vi "Ass IO Status.vi"(8 "error in (no error)":errorcluster) -> (0 "error out":errorcluster)   [LabVIEW 2017]
uses:
  <vilib>/NI/Modbus Library/API/Wrapper/Create TCP Master.vi
  <vilib>/NI/Modbus Library/API/master/Modbus Master.lvclass
  <vilib>/NI/Modbus Library/API/Wrapper/API Main.lvlib
panel:
  in  "Tab Control":enum32{"INPUTS", "OUTPUTS"}(tab)
  out "Cycle Start-1":bool
  out "Cycle Start-2":bool
  out "Reset":bool
  out "Emergency":bool
  out "Bin-1":bool
  out "Bin-2":bool
  out "Bin-3":bool
  out "Bin-4":bool
  out "Bin-5":bool
  out "Bin-6":bool
  out "Bin-7":bool
  out "Bin-8":bool
  out "Part Presence":bool
  out "OK Cam-1":bool
  out "NOK Cam-1":bool
  out "OK Cam-2":bool
  out "NOK Cam-2":bool
  out "Part Clamp Fwd":bool
  out "Part Clamp Rev":bool
  in  "Red Tower Lamp":bool
  in  "Buzzer Tower Lamp":bool
  in  "Yellow Tower Lamp":bool
  in  "Green Tower Lamp":bool
  in  "Orange Ind Bin-01":bool
  in  "Yellow Ind Bin-01":bool
  in  "Green Ind Bin-01":bool
  in  "Orange Ind Bin-02":bool
  in  "Yellow Ind Bin-02":bool
  in  "Green Ind Bin-02":bool
  in  "Yellow Ind Bin-03":bool
  in  "Green Ind Bin-03":bool
  in  "Orange Ind Bin-04":bool
  in  "Yellow Ind Bin-04":bool
  in  "Green Ind Bin-04":bool
  in  "Orange Ind Bin-05":bool
  in  "Yellow Ind Bin-05":bool
  in  "Green Ind Bin-05":bool
  in  "Orange Ind Bin-06":bool
  in  "Yellow Ind Bin-06":bool
  in  "Orange Ind Bin-07":bool
  in  "Yellow Ind Bin-07":bool
  in  "Green Ind Bin-07":bool
  in  "Orange Ind Bin-08":bool
  in  "Yellow Ind Bin-08":bool
  in  "Green Ind Bin-08":bool
  in  "Clamping Cylinder":bool
  in  "Start Trigger Cam-1":bool
  in  "Start Trigger Cam-2":bool
  in  "Spare-1":bool
  in  "Orange Ind Bin-03":bool
  in  "Green Ind Bin-06":bool
  in  "Spare-2":bool
  in  "stop":bool
  # "ASSEMBLY STATION IO STATUS"
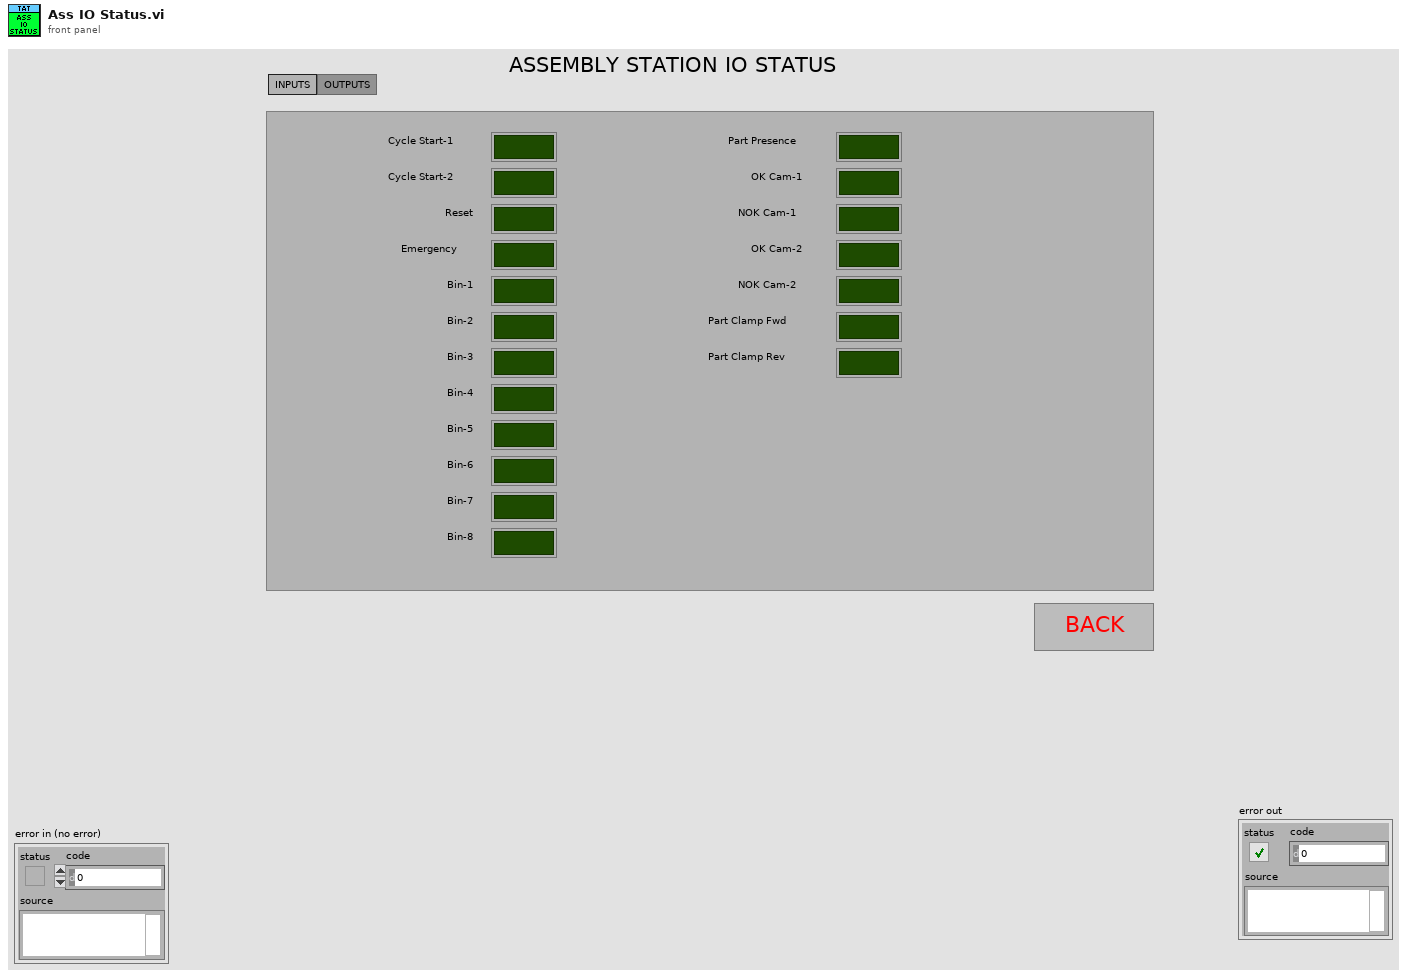
[diagram p1: front panel]
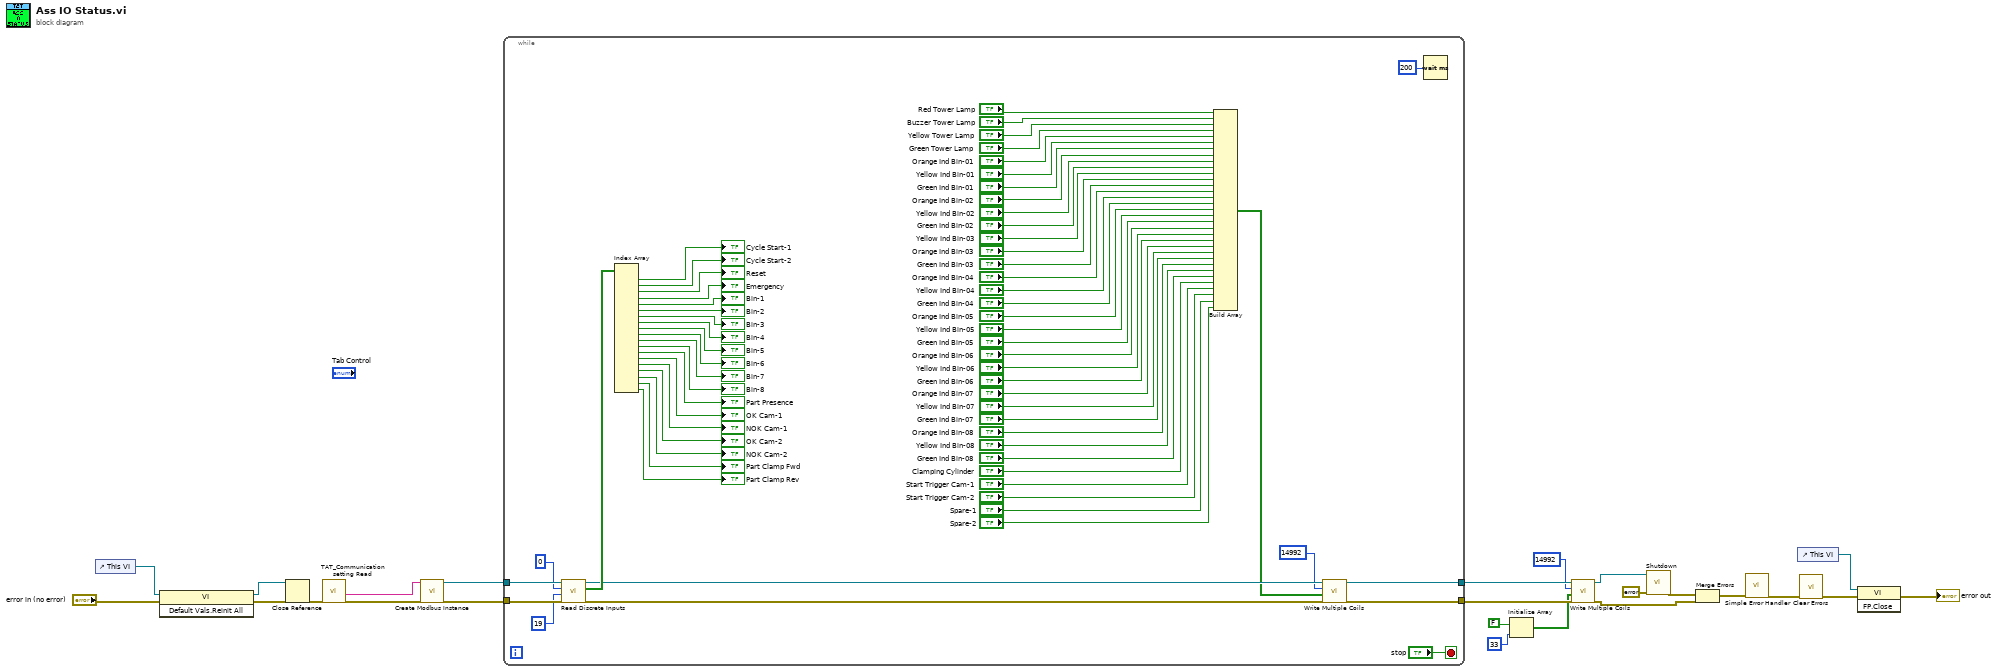
[diagram p0: block diagram]
diagram:
  n1 = control-ref of="This VI"() -> (w5:refnum<vi>)
  n2 = invoke class="VI" method="Default Vals.Reinit All"(reference=w5, error in="error in (no error)") -> (reference out=w3:refnum<vi>, error out=w2:errorcluster)  [unwired: 1 in, 1 out]
  n3 = Close Reference(reference=w3, error in (no error)=w2) -> (error out=w1:errorcluster)
  n4 = call "TAT_Communication setting Read.vi"("error in (no error)"=w1) -> ("error out"=w24:errorcluster, "PLC IP"=w23:string)  [unwired: 3 in, 6 out]
  n5 = call-poly <vilib>:"Create Modbus Instance.vi"("error in"=w24, "address"=w23) -> ("error out"=w22:errorcluster, "TCP master instance"=w21:refnum<class "Modbus Master.lvclass">)  [unwired: 8 in]
  n6 = while {
    tunnel: w22 -> [w88]
    tunnel: w21 -> [w87]
    tunnel: [w26] -> w11
    tunnel: [w25] -> w13
    stop <- "stop" stop-if-true
    n7 = call-dynamic "Read Discrete Inputs.vi"("error in"=w88, "number of inputs"=u16 19, "starting address"=u16 0, "Modbus master in"=w87) -> ("error out"=w62:errorcluster, "discrete inputs"=w84:bool[], "Modbus master out"=w63:refnum<class "Modbus Master.lvclass">)  [unwired: 5 in]
    n8 = Index Array(array=w84) -> (element #1=→"Cycle Start-1":bool, element #2=→"Cycle Start-2":bool, element #3=→"Reset":bool, element #4=→"Emergency":bool, element #5=→"Bin-1":bool, element #6=→"Bin-2":bool, element #7=→"Bin-3":bool, element #8=→"Bin-4":bool, element #9=→"Bin-5":bool, element #10=→"Bin-6":bool, element #11=→"Bin-7":bool, element #12=→"Bin-8":bool, element #13=→"Part Presence":bool, element #14=→"OK Cam-1":bool, element #15=→"NOK Cam-1":bool, element #16=→"OK Cam-2":bool, element #17=→"NOK Cam-2":bool, element #18=→"Part Clamp Fwd":bool, element #19=→"Part Clamp Rev":bool)  [unwired: 19 in]
    n9 = Build Array("Red Tower Lamp", "Buzzer Tower Lamp", "Yellow Tower Lamp", "Green Tower Lamp", "Orange Ind Bin-01", "Yellow Ind Bin-01", "Green Ind Bin-01", "Orange Ind Bin-02", "Yellow Ind Bin-02", "Green Ind Bin-02", "Yellow Ind Bin-03", "Orange Ind Bin-03", "Green Ind Bin-03", "Orange Ind Bin-04", "Yellow Ind Bin-04", "Green Ind Bin-04", "Orange Ind Bin-05", "Yellow Ind Bin-05", "Green Ind Bin-05", "Orange Ind Bin-06", "Yellow Ind Bin-06", "Green Ind Bin-06", "Orange Ind Bin-07", "Yellow Ind Bin-07", "Green Ind Bin-07", "Orange Ind Bin-08", "Yellow Ind Bin-08", "Green Ind Bin-08", "Clamping Cylinder", "Start Trigger Cam-1", "Start Trigger Cam-2", "Spare-1", "Spare-2") -> (w27:bool[])
    n10 = call-dynamic "Write Multiple Coils.vi"("error in"=w62, "coils to write"=w27, "starting address"=u16 14992, "Modbus master in"=w63) -> ("error out"=w26:errorcluster, "Modbus master out"=w25:refnum<class "Modbus Master.lvclass">)  [unwired: 6 in]
    n11 = Wait (ms)(milliseconds to wait=u32 200) -> ()  [unwired: 1 out]
  }
  n12 = Initialize Array(FALSE, 33 ("dimension size")) -> (w6:bool[])
  n13 = call-dynamic "Write Multiple Coils.vi"("error in"=w11, "coils to write"=w6, "starting address"=u16 14992, "Modbus master in"=w13) -> ("error out"=w10:errorcluster, "Modbus master out"=w12:refnum<class "Modbus Master.lvclass">)  [unwired: 6 in]
  n14 = call-dynamic "Shutdown.vi"("error in"=errorcluster {"status"=FALSE, "code"=0, "source"=""}, "Modbus master in"=w12) -> ("error out"=w19:errorcluster)  [unwired: 9 in]
  n15 = Merge Errors(w19, w10) -> (w18:errorcluster)
  n16 = call <vilib>:"Simple Error Handler.vi"("error in (no error)"=w18) -> ("error out"=w17:errorcluster)  [unwired: 4 in, 4 out]
  n17 = control-ref of="This VI"() -> (w15:refnum<vi>)
  n18 = call <vilib>:"Clear Errors.vi"("error in (no error)"=w17) -> ("error out"=w16:errorcluster)  [unwired: 5 in, 1 out]
  n19 = invoke class="VI" method="FP.Close"(reference=w15, error in=w16) -> (error out=→"error out":errorcluster)  [unwired: 1 in, 2 out]
